vi "ADAM 5000 Get Voltages - 12Bit.vi"(8 "error in (no error)":errorcluster, 9 "Bd # (0=first bd)":u16, 11 "Remote IP Address 2":string="192.168.0.200") -> (0 "error out":errorcluster, 1 "Slave Input Registers 2":u16[](array[numeric])=[38065, 32770, 32770, 32767, 32770, 32767, 32767, 32767] caption="Slave Input Registers (Read Only)", 2 "Data":dbl[](array[numeric])=[0.7972994999999994, -0.009129000000000609, -0.009129000000000609, -0.009585900000000258, -0.009129000000000609, -0.009585900000000258, -0.009585900000000258, -0.009585900000000258])   [LabVIEW 2014, in "UI Core.lvlib"]
uses:
  VIs/UI Core.lvlib
  nimodbus121/71/vi.lib/NI Modbus.llb/MB Modbus Command.ctl
panel:
  in  "Modbus Command":T1={"Function Code"=3, "Starting Address"=0, "Quantity"=8, "Data"=[], "Discrete"=[]} {"Function Code" items=["Read Coils"=1, "Read Discrete Inputs"=2, "Read Holding Registers"=3, "Read Input Registers"=4, "Write Single Coil"=5, "Write Single Register"=6, "Read Exception Status"=7, "Write Multiple Coils"=15, "Write Multiple Registers"=16]}
  in  "Remote Port 2":u16=502
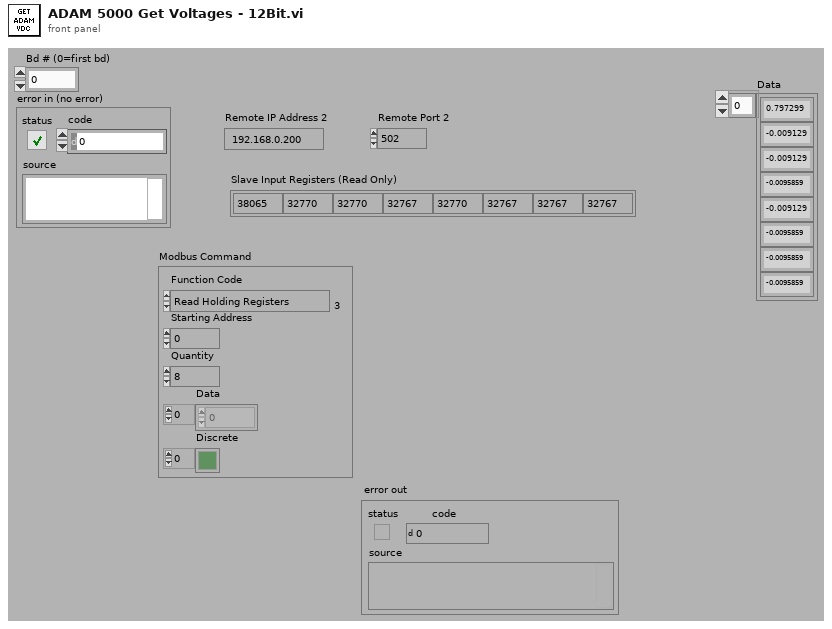
[diagram p1: front panel]
types:
  T1 = typedef "MB Modbus Command.ctl" = cluster{"Function Code":u8, "Starting Address":u16, "Quantity":u16, "Data":u16[], "Discrete":bool[]}
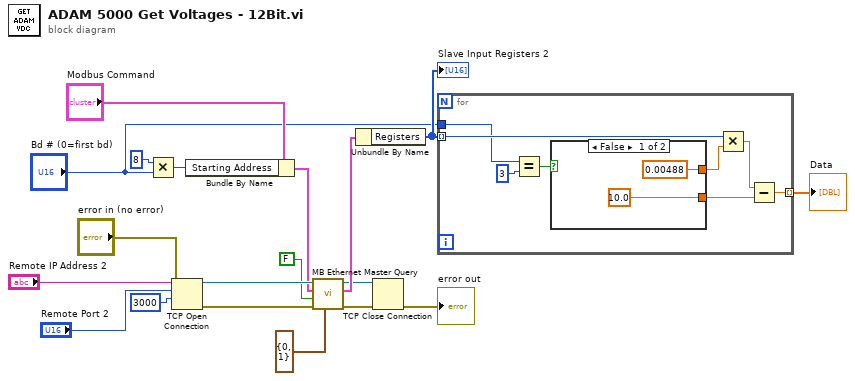
[diagram p0: block diagram]
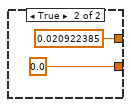
[diagram p2: hidden frame]
diagram:
  n1 = Multiply(x=u16 8, y="Bd # (0=first bd)") -> (x*y=w7:u16)
  n2 = TCP Open Connection(address="Remote IP Address 2", remote port or service name="Remote Port 2", timeout ms (60000)=3000, error in (no error)="error in (no error)") -> (connection ID=w17:refnum<k5>, error out=w4:errorcluster)  [unwired: 1 in]
  n3 = Bundle By Name(cluster="Modbus Command", "Starting Address"=w7) -> (w6:T1)
  n4 = call "MB Ethernet Master Query.vi"("MBAP Header"=cluster{"Transaction ID":u16, "Unit ID":u8} {"Transaction ID"=0, "Unit ID"=1}, "error in (no error)"=w4, "Use MODBUS Data Unit?"=FALSE, "Modbus Command"=w6, "TCP Connection Refnum in"=w17) -> ("error out"=w3:errorcluster, "Registers"=w15:cluster{"Registers":u16[], "Discrete":bool[]}, "TCP Connection Refnum (dup)"=w10:refnum<k5>)  [unwired: 2 in, 2 out]
  n5 = Unbundle By Name(w15) -> ("Registers"=w12:u16[])
  "Slave Input Registers 2" <- w12
  n6 = TCP Close Connection(connection ID=w10, error in (no error)=w3) -> (error out=→"error out":errorcluster)  [unwired: 1 in, 1 out]
  n7 = for {
    tunnel: w12 -> [w27] mode=indexing
    tunnel: [w23] -> w11 mode=indexing
    tunnel: "Bd # (0=first bd)" -> [w21]
    n8 = Equal?(x=w21, y=u16 3) -> (x = y?=w22:bool)
    n9 = case shown="False" w22 {
      tunnel: [0.00488 ("y") 0.020922385 ("y")] -> w26
      tunnel: [10.0 ("y") 0.0 ("y")] -> w24
      frame False {
      }
      frame True {
      }
    }
    n10 = Multiply(x=w27, y=w26) -> (x*y=w25:dbl)
    n11 = Subtract(x=w25, y=w24) -> (x-y=w23:dbl)
  }
  "Data" <- w11
